vi "Read Package Data.vi"(8 "error in (no error)":errorcluster, 11 "DataContainer in":refnum<class "DataContainer.lvclass">) -> (0 "error out":errorcluster, 2 "Package Data":T1[](array[typedef]) {"payload" format="%x"; "timestamp" format="%<%.7X\n%x>T"; "type" items=["FlexRay Data"=32, "FlexRay Null"=33, "FlexRay Symbol"=34, "Log Trigger"=225, "Start Trigger"=226]; "cycle count" max=63 step=1}, 3 "DataContainer out":refnum<class "DataContainer.lvclass">)   [LabVIEW 2023, in "DataContainer.lvclass"]
uses:
  DataContainer.lvclass
  <vilib>/xnet/xnet.llb/XNET Frame FlexRay.ctl
  <vilib>/xnet/xnet.llb/XNET Frame Type FlexRay.ctl
  DataContainer.lvclass/DataContainer.ctl
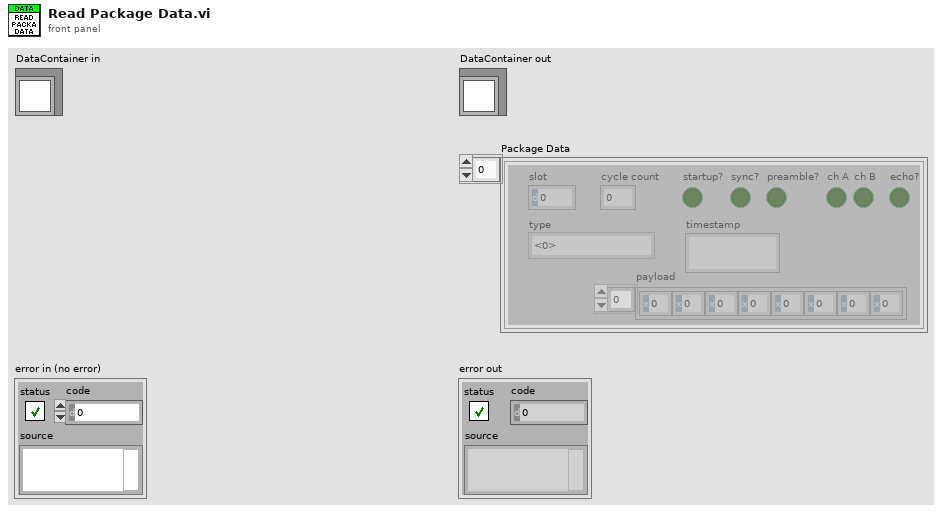
[diagram p1: front panel]
types:
  T1 = typedef "XNET Frame FlexRay.ctl" = cluster{"timestamp":timestamp, "payload":u8[], "slot":u16, "type":T2, "cycle count":u8, "startup?":bool, "sync?":bool, "preamble?":bool, "ch A":bool, "ch B":bool, "echo?":bool}
  T2 = typedef "XNET Frame Type FlexRay.ctl" = u8
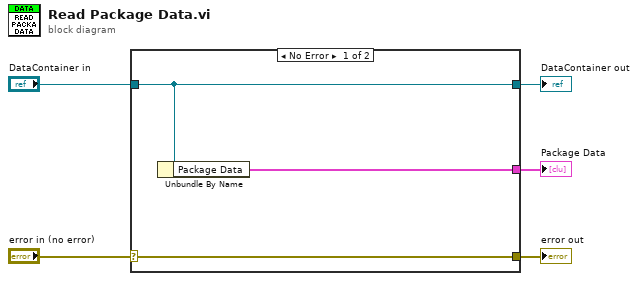
[diagram p0: block diagram]
diagram:
  n1 = case shown="No Error" "error in (no error)" {
    selector: "error in (no error)" -> [w8 w9]
    tunnel: [w8 w9] -> w4
    tunnel: [w7 w10] -> w2
    tunnel: "DataContainer in" -> [w7 w10]
    tunnel: [w6 _] -> w1
    frame No Error {
      n2 = Unbundle By Name(w7) -> ("Package Data"=w6:T1[])
    }
    frame Error {
    }
  }
  "error out" <- w4
  "DataContainer out" <- w2
  "Package Data" <- w1
